vi "DELETE THIS Get DAQChannel Info.vi"(8 "error in (no error)":errorcluster, 11 "Sequencer in":refnum<class "Sequencer.lvclass">) -> (0 "error out":errorcluster, 3 "Sequencer out":refnum<class "Sequencer.lvclass">)   [LabVIEW 2015, in "Sequencer.lvlib" / "Sequencer.lvclass"]
uses:
  Sequencer.lvclass
  <resource>/objmgr/daqmx.rc
  SequencerInfo.lvclass
  SequencerConfig.lvclass
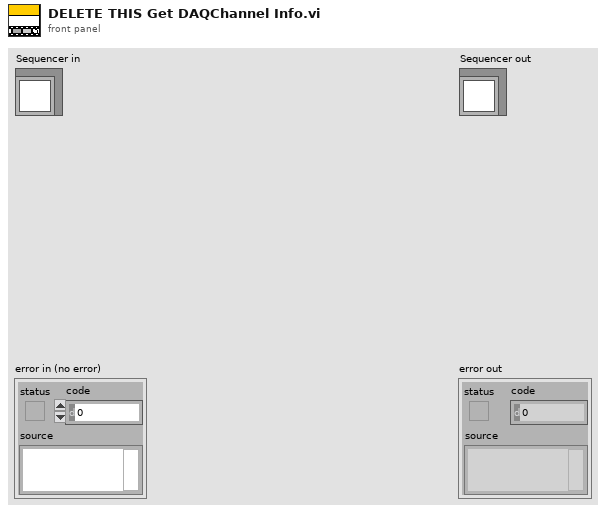
[diagram p1: front panel]
types:
  T1 = typedef "Sequencer.lvlib/Sequencer.lvclass/Daq Channel Info.ctl" = cluster{"DevNames":tag[], "AO.PhysicalChans":tag[][], "DO.Lines":tag[][], "AI.PhysicalChans":tag[][]}
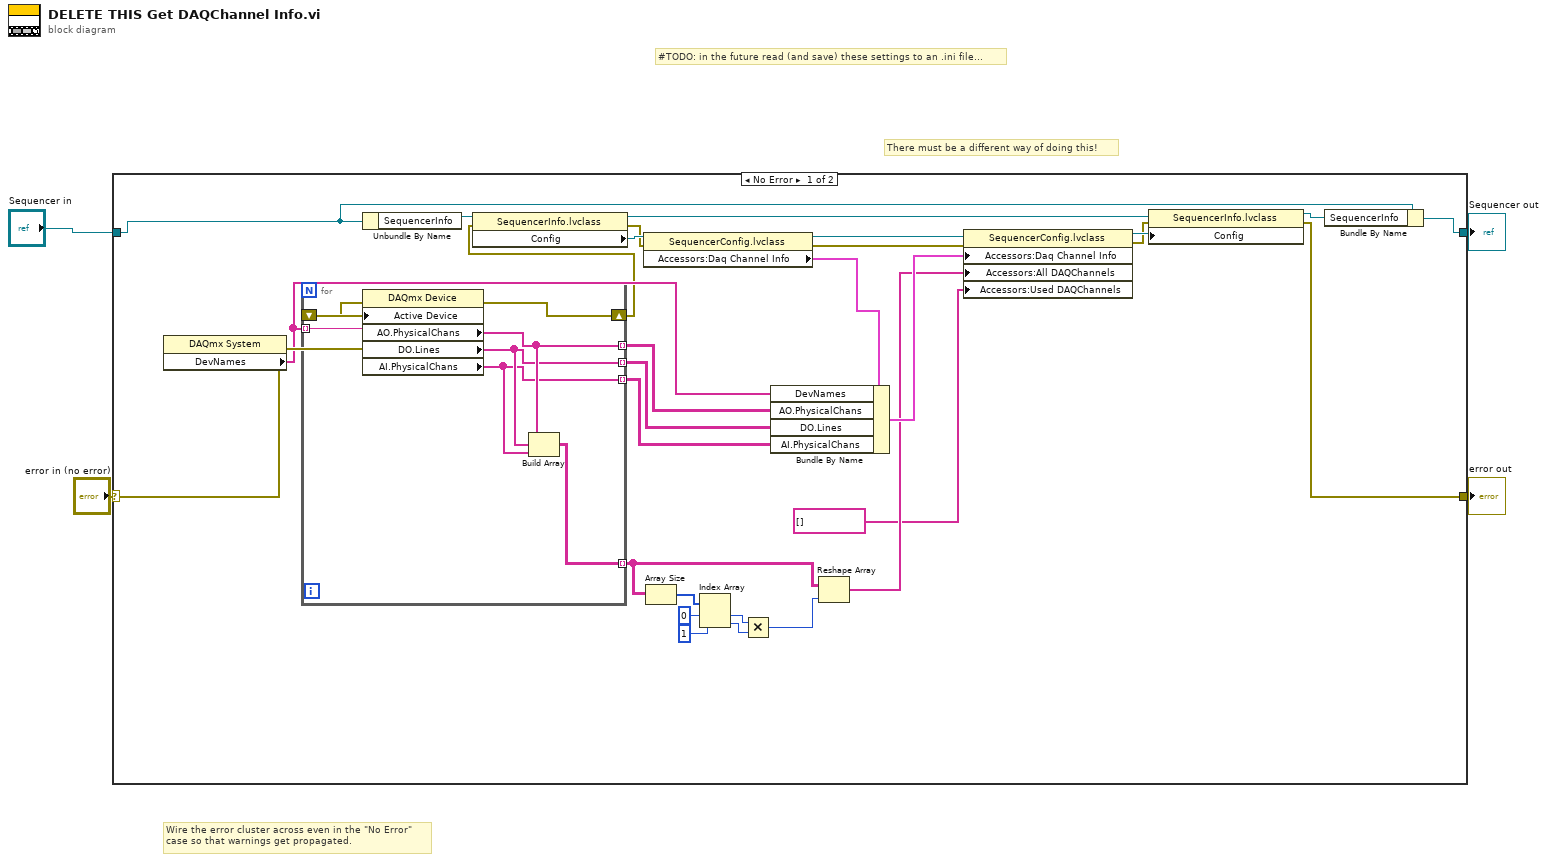
[diagram p0: block diagram]
diagram:
  # "There must be a different way of doing this!"
  # "Wire the error cluster across even in the \"No Error\"\ncase so that warnings get propagated."
  # "#TODO: in the future read (and save) these settings to an .ini file..."
  n1 = case shown="No Error" "error in (no error)" {
    selector: "error in (no error)" -> [w29 w43]
    tunnel: [w8 w43] -> w3
    tunnel: [w13 w42] -> w1
    tunnel: "Sequencer in" -> [w15 w42]
    frame No Error {
      n2 = property class="DAQmx System"(error in=w29) -> (error out=w34:errorcluster, "DevNames"=w33:tag[])  [unwired: 1 in, 1 out]
      n3 = for {
        tunnel: w33 -> [w41] mode=indexing
        tunnel: [w38] -> w30 mode=indexing
        tunnel: [w37] -> w31 mode=indexing
        tunnel: [w36] -> w32 mode=indexing
        shift-right: [w39] -> w11
        shift-left: w34 -> [w40]
        tunnel: [w35] -> w23 mode=indexing
        n4 = property class="DAQmx Device"(error in=w40, "Active Device"=w41) -> (error out=w39:errorcluster, "AO.PhysicalChans"=w38:tag[], "DO.Lines"=w37:tag[], "AI.PhysicalChans"=w36:tag[])  [unwired: 1 in, 1 out]
        n5 = Build Array(w38, w37, w36) -> (w35:tag[][])
      }
      n6 = Unbundle By Name(w15) -> ("SequencerInfo"=w21:refnum<class "SequencerInfo.lvclass">)
      n7 = property class="SequencerInfo.lvclass"(reference=w21, error in=w11) -> (reference out=w7:refnum<class "SequencerInfo.lvclass">, error out=w10:errorcluster, "Config"=w20:refnum<class "SequencerConfig.lvclass">)
      n8 = property class="SequencerConfig.lvclass"(reference=w20, error in=w10) -> (reference out=w5:refnum<class "SequencerConfig.lvclass">, error out=w9:errorcluster, "Accessors:Daq Channel Info"=w19:T1)
      n9 = Array Size(array=w23) -> (size(s)=w28:i32[])
      n10 = Index Array(array=w28, index #1=0 ("index"), index #2=1 ("index")) -> (element #1=w25:i32, element #2=w24:i32)
      n11 = Multiply(x=w25, y=w24) -> (x*y=w22:i32)
      n12 = Bundle By Name(cluster=w19, "DevNames"=w33, "AO.PhysicalChans"=w30, "DO.Lines"=w31, "AI.PhysicalChans"=w32) -> (w18:T1)
      n13 = Reshape Array(w23, w22) -> (w17:tag[])
      n14 = property class="SequencerConfig.lvclass"(reference=w5, error in=w9, "Accessors:Daq Channel Info"=w18, "Accessors:All DAQChannels"=w17, "Accessors:Used DAQChannels"=tag[] [] ("Used DAQChannels")) -> (reference out=w16:refnum<class "SequencerConfig.lvclass">, error out=w6:errorcluster)
      n15 = property class="SequencerInfo.lvclass"(reference=w7, error in=w6, "Config"=w16) -> (reference out=w14:refnum<class "SequencerInfo.lvclass">, error out=w8:errorcluster)
      n16 = Bundle By Name(cluster=w15, "SequencerInfo"=w14) -> (w13:refnum<class "Sequencer.lvclass">)
    }
    frame Error {
    }
  }
  "error out" <- w3
  "Sequencer out" <- w1
